vi "DSF.Execution.Builder.Set Framework Cache.vi"(8 "error in (no error)":errorcluster, 10 "Framework Cache":refnum<class "DSF.Engine.Memory.Cache.Framework.lvclass">, 11 "Builder in":refnum<class "DSF.Execution.Builder.lvclass">) -> (0 "error out":errorcluster, 3 "Builder out":refnum<class "DSF.Execution.Builder.lvclass">)   [LabVIEW 2016, in "DSF.Engine.lvlib" / "DSF.Execution.Builder.lvclass"]
uses:
  DSF.Execution.Builder.lvclass
  Memory.Cache/DSF.Engine.Memory.Cache.Framework.lvclass
  DSF.Execution.Builder.lvclass/DSF.Execution.Builder.ctl
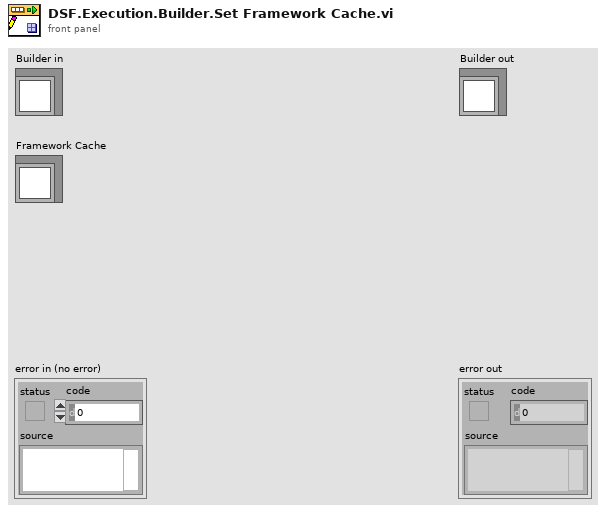
[diagram p1: front panel]
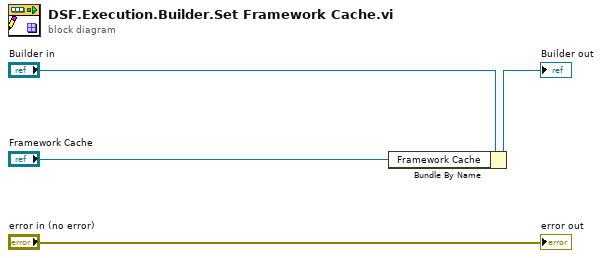
[diagram p0: block diagram]
diagram:
  n1 = Bundle By Name(cluster="Builder in", "Framework Cache"="Framework Cache") -> (→"Builder out":refnum<class "DSF.Execution.Builder.lvclass">)
  "error out" <- "error in (no error)"
